vi "SRI8610C-CheckForFileUpdate.vi"(7 "State":T1=enum."Run", 8 "error in":errorcluster) -> (0 "error out":errorcluster, 2 "File Updated?":bool, 4 "Elapsed Time Since Last Update (sec)":dbl)   [LabVIEW 2023, in "SRI8610C-GasChromatograph.lvlib"]
uses:
  SRI8610C-GasChromatograph.lvlib
  Controls/SRI8610C-States-InitRun.ctl
panel:
  out "last mod":timestamp
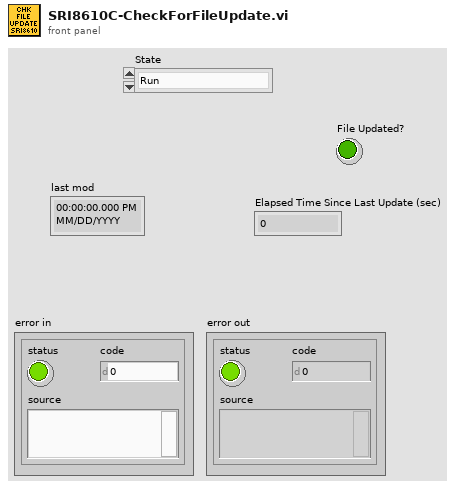
[diagram p1: front panel]
types:
  T1 = typedef "SRI8610C-States-InitRun.ctl" = enum16{"Initialize", "Run"}
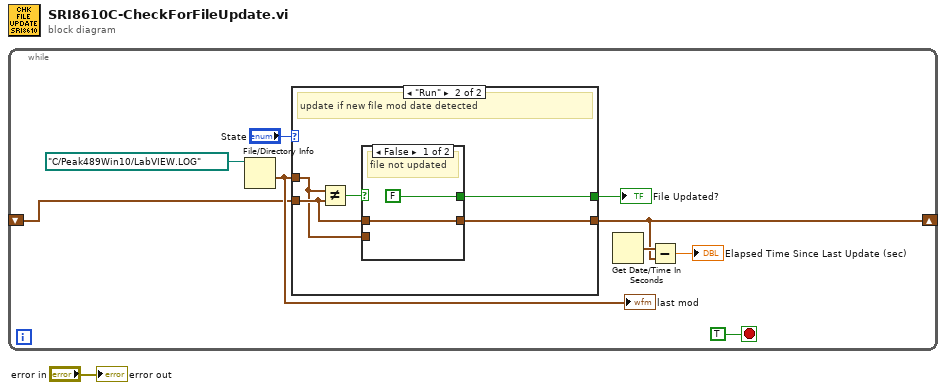
[diagram p0: block diagram]
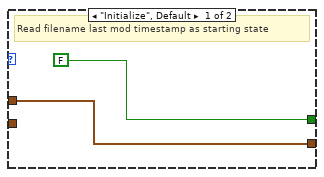
[diagram p2: hidden frame]
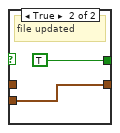
[diagram p3: hidden frame]
diagram:
  n1 = while {
    shift-right: [w3] -> _
    shift-left: _ -> [w6]
    stop <- TRUE stop-if-true
    n2 = File/Directory Info(path=path "C:/Peak489Win10/LabVIEW.LOG" ("file (use dialog)")) -> (last mod=w7:timestamp)  [unwired: 1 in, 6 out]
    "last mod" <- w7
    n3 = case shown="\"Run\"" "State" {
      tunnel: w7 -> [w12 w14]
      tunnel: [w12 w16] -> w3
      tunnel: w6 -> [_ w15]
      tunnel: [FALSE w13] -> w5
      frame "Initialize", Default {
        # "Read filename last mod timestamp as starting state"
      }
      frame "Run" {
        # "update if new file mod date detected"
        n4 = Not Equal?(x=w14, y=w15) -> (x != y?=w17:bool)
        n5 = case shown="False" w17 {
          tunnel: [w19 w21] -> w16
          tunnel: w15 -> [w19 _]
          tunnel: w14 -> [_ w21]
          tunnel: [FALSE TRUE] -> w13
          frame False {
            # "file not updated"
          }
          frame True {
            # "file updated"
          }
        }
      }
    }
    "File Updated?" <- w5
    n6 = Get Date/Time In Seconds() -> (seconds since 1Jan1904=w4:timestamp)
    n7 = Subtract(x=w4, y=w3) -> (x-y=→"Elapsed Time Since Last Update (sec)":dbl)
  }
  "error out" <- "error in"
